vi "zero all phys units.vi"(4 "zero interval (s)":dbl=1.0 min=1.0 format="%.1f", 5 "Data frequency":ext=1.0 format="%.2f", 6 "History Data":sgl[][](array[numeric]) format="%.2f") -> ()   [LabVIEW 2012]
uses:
  <vilib>/Analysis/baseanly.llb/Mean (DBL).vi
  <vilib>/Analysis/NI_AALBase.lvlib
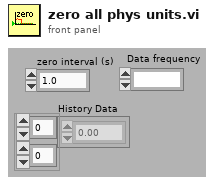
[diagram p1: front panel]
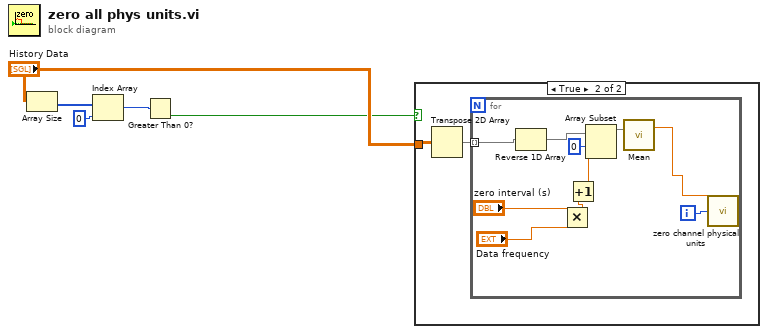
[diagram p0: block diagram]
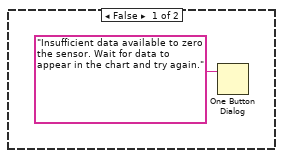
[diagram p2: hidden frame]
diagram:
  n1 = Array Size(array="History Data") -> (size(s)=w4:i32[])
  n2 = Index Array(array=w4, index=0) -> (element=w1:i32)
  n3 = Greater Than 0?(x=w1) -> (x > 0?=w3:bool)
  n4 = case shown="True" w3 {
    tunnel: "History Data" -> [_ w8]
    frame False {
      n5 = One Button Dialog(message="Insufficient data available to zero the sensor. Wait for data to appear in the chart and try again.") -> ()  [unwired: 1 in, 1 out]
    }
    frame True {
      n6 = Transpose 2D Array(2D array=w8) -> (transposed array=w7:sgl[][])
      n7 = for {
        tunnel: w7 -> [w11] mode=indexing
        i -> [w9]
        n8 = Reverse 1D Array(array=w11) -> (reversed array=w17:sgl[])
        n9 = Multiply(x="zero interval (s)", y="Data frequency") -> (x*y=w14:ext)
        n10 = Increment(x=w14) -> (x+1=w12:ext)
        n11 = Array Subset(array=w17, index=0, length=w12) -> (w18:sgl[])
        n12 = call-poly <vilib>:"Mean.vi"("X"=w18) -> ("mean"=w10:dbl)  [unwired: 1 out]
        n13 = call "zero channel physical units.vi"("Index"=w9, "Mean (physical units)"=w10) -> ()  [unwired: 6 in]
      }
    }
  }
